vi "Create Channels from Parameter List (RT).vi"(7 "Message Param map in":T1, 8 "error in (no error)":errorcluster, 10 "Param ID map in":map{i32, string}(c390), 11 "channel ref in":T2=18446744073709551615 format="%.0x") -> (0 "error out":errorcluster, 2 "Param ID map out":map{i32, string}(c390), 3 "channel ref out":T2=18446744073709551615 format="%.0x", 5 "Message Param map out":T1)   [LabVIEW 2020, in "Ballard 1553 System Explorer.lvlib"]
uses:
  Ballard 1553 System Explorer.lvlib
  <vilib>/NI VeriStand/Custom Device API/Custom Device Item Ref.ctl
  Parse XML Ballard/Ballard_RT direction.ctl
  <vilib>/NI VeriStand/Custom Device API/Custom Device Channel Type.ctl
  Shared/Controls and Global/Global.vi
  <vilib>/NI VeriStand/Custom Device Tools/Custom Device Utility Library/NI VeriStand - Search for All Items by GUID.vi
  <vilib>/NI VeriStand/Custom Device API/Get Item Property (I32).vi
  <vilib>/NI VeriStand/Custom Device API/Get Item Property (U16).vi
  <vilib>/NI VeriStand/Custom Device Tools/Custom Device Utility Library/NI VeriStand - Search for Item by GUID.vi
  <vilib>/NI VeriStand/Custom Device Tools/Custom Device Utility Library/Custom Device Utility Library.lvlib
  Shared/Ballard 1553 Shared.lvlib
  <vilib>/NI VeriStand/Custom Device API/Custom Device API.lvlib
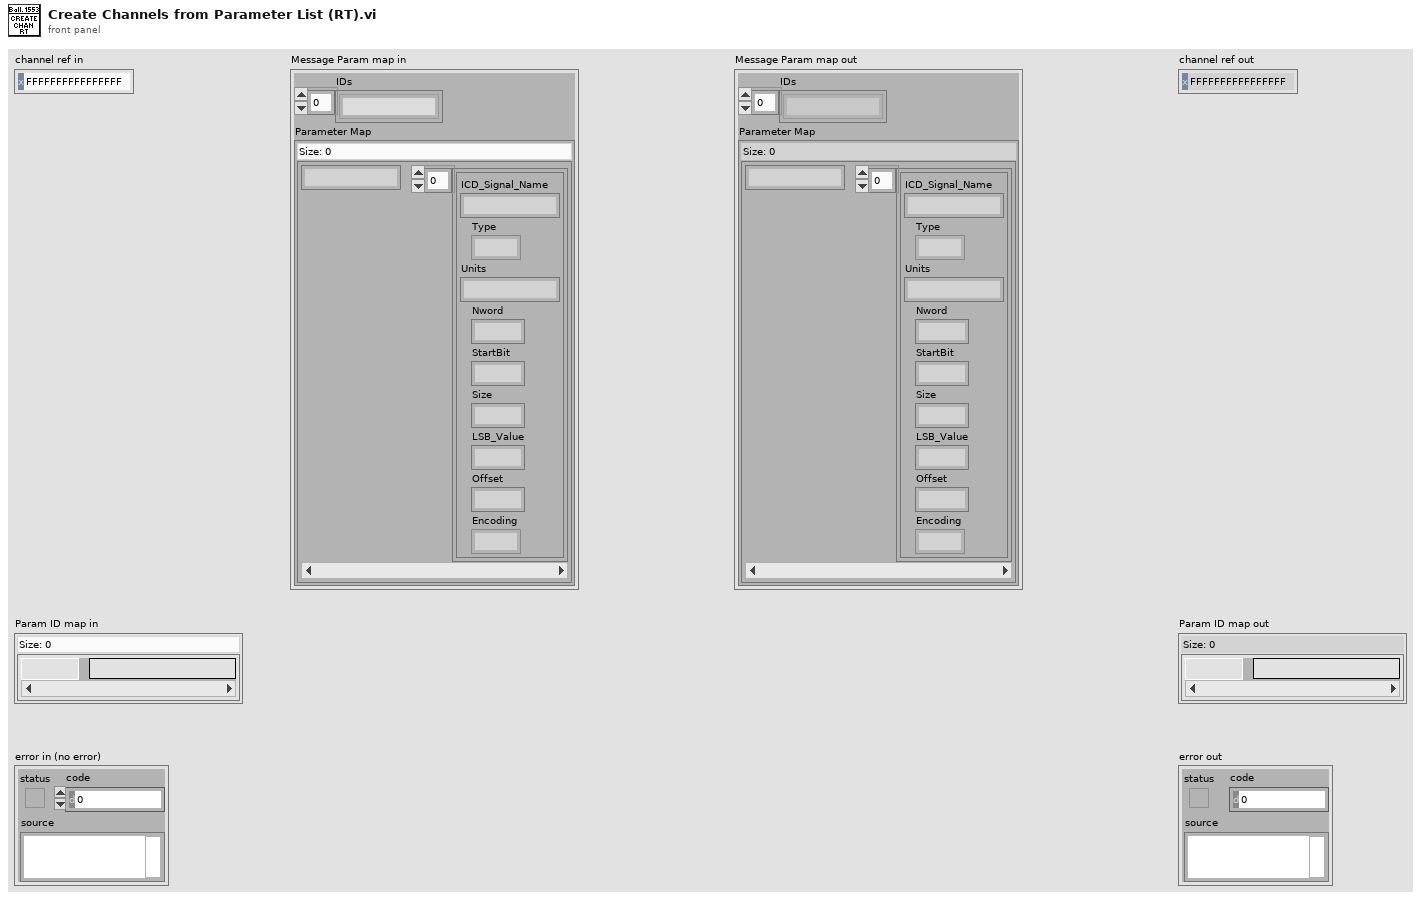
[diagram p1: front panel]
types:
  T1 = cluster{"IDs":string[], "Parameter Map":map{string, cluster{"ICD_Signal_Name":string, "Type":enum16{"Opaque", "Enum", "Float", "Integer", "Bcd", "Bool"}, "Units":string, "Nword":i32, "StartBit":i32, "Size":i32, "LSB_Value":dbl, "Offset":i32, "Encoding":enum16{"None", "2-complement", "Unsigned"}}[]}}
  T2 = typedef "Custom Device API.lvlib/Custom Device Item Ref.ctl" = u64
  T3 = typedef "Ballard 1553 System Explorer.lvlib/Ballard_RT direction.ctl" = enum16{"Tx", "Rx"}
  T4 = typedef "Custom Device API.lvlib/Custom Device Channel Type.ctl" = enum16{"Input", "Output"}
  T5 = map{string, cluster{"ICD_Signal_Name":string, "Type":enum16{"Opaque", "Enum", "Float", "Integer", "Bcd", "Bool"}, "Units":string, "Nword":i32, "StartBit":i32, "Size":i32, "LSB_Value":dbl, "Offset":i32, "Encoding":enum16{"None", "2-complement", "Unsigned"}}[]}
  T6 = cluster{"ICD_Signal_Name":string, "Type":enum16{"Opaque", "Enum", "Float", "Integer", "Bcd", "Bool"}, "Units":string, "Nword":i32, "StartBit":i32, "Size":i32, "LSB_Value":dbl, "Offset":i32, "Encoding":enum16{"None", "2-complement", "Unsigned"}}[]
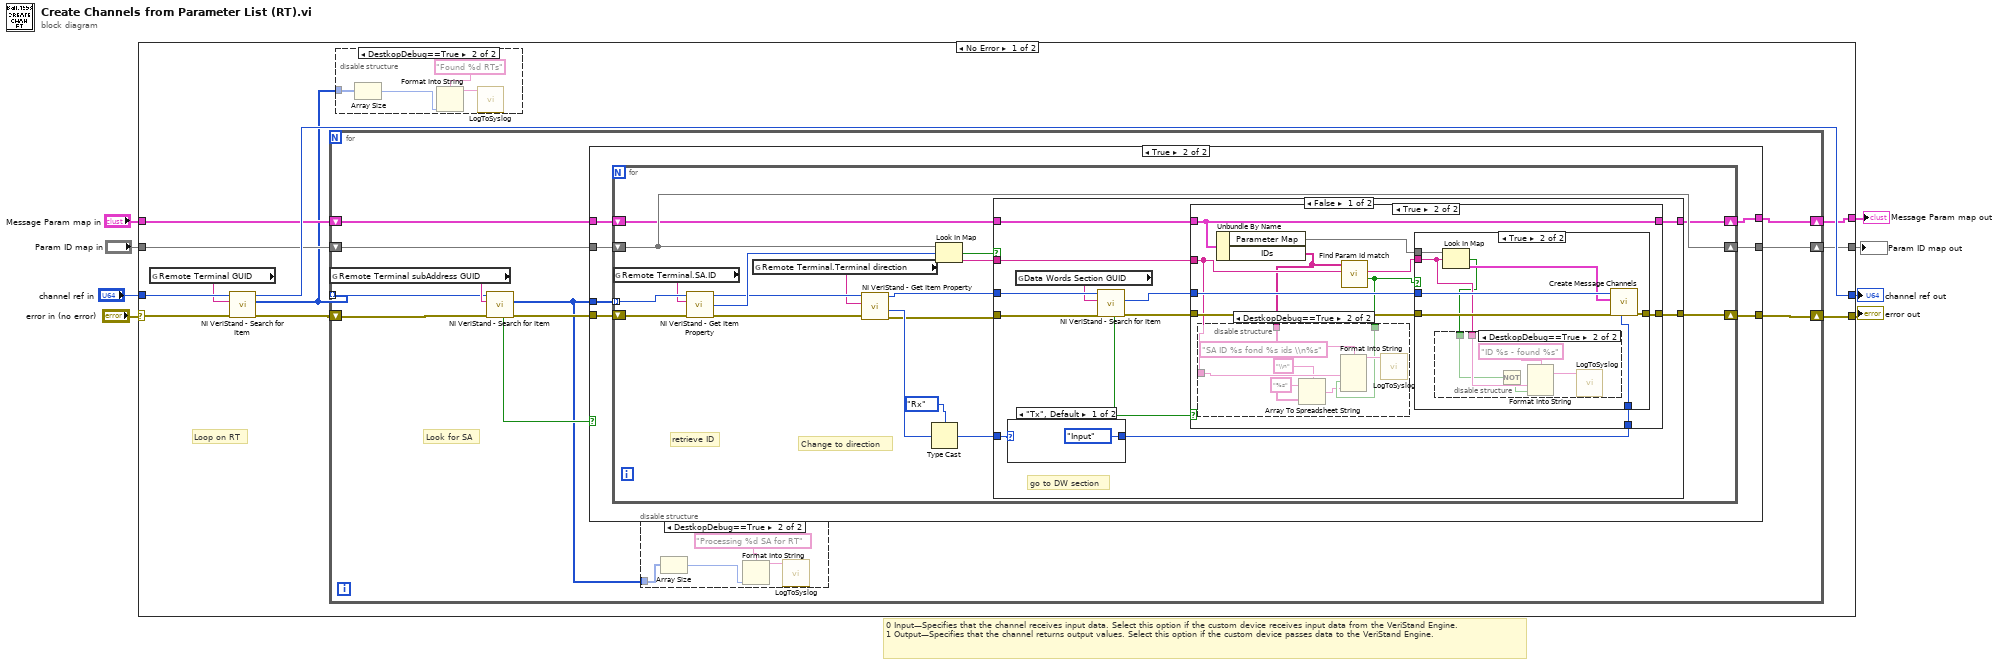
[diagram p0: block diagram]
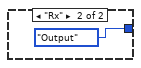
[diagram p4: hidden frame]
diagram:
  # "0 Input—Specifies that the channel receives input data. Select this option if the custom device receives input data from the VeriStand Engine. \n1 Output—Specifies that the channel returns output values. Select this option if the custom device passes data to the VeriStand Engine."
  n1 = case shown="No Error" "error in (no error)" {
    selector: "error in (no error)" -> [w18 w118]
    tunnel: "channel ref in" -> [w19 w120]
    tunnel: "Param ID map in" -> [w14 w119]
    tunnel: [w17 w120] -> w5
    tunnel: [w13 w119] -> w4
    tunnel: [w15 w118] -> w3
    tunnel: "Message Param map in" -> [w12 w117]
    tunnel: [w11 w117] -> w1
    frame No Error {
      # "Loop on RT"
      n2 = global read "Global.vi" "Remote Terminal GUID"() -> (w10:string)
      n3 = call-poly <vilib>:"NI VeriStand - Search for Item.vi"("error in"=w18, "Item GUID"=w10, "Section Ref in"=w19) -> ("error out"=w16:errorcluster, "Item Refs"=w9:T2[], "Section Ref out"=w17:T2)  [unwired: 5 in, 1 out]
      n4 = for {
        tunnel: w9 -> [w25] mode=indexing
        shift-right: [w27] -> w15
        shift-left: w16 -> [w30]
        shift-right: [w21] -> w11
        shift-left: w12 -> [w22]
        shift-right: [w23] -> w13
        shift-left: w14 -> [w24]
        # "Look for SA"
        n5 = global read "Global.vi" "Remote Terminal subAddress GUID"() -> (w29:string)
        n6 = call-poly <vilib>:"NI VeriStand - Search for Item.vi"("error in"=w30, "Item GUID"=w29, "Section Ref in"=w25) -> ("error out"=w26:errorcluster, "Item Refs"=w20:T2[], "Found"=w28:bool)  [unwired: 5 in, 1 out]
        n7 = case shown="True" w28 {
          tunnel: w20 -> [_ w44]
          tunnel: [w37 w42] -> w27
          tunnel: w26 -> [w37 w43]
          tunnel: w24 -> [w36 w41]
          tunnel: [w36 w40] -> w23
          tunnel: w22 -> [w35 w39]
          tunnel: [w35 w38] -> w21
          frame False {
          }
          frame True {
            n8 = for {
              tunnel: w44 -> [w60] mode=indexing
              shift-right: [w62] -> w42
              shift-left: w43 -> [w61]
              shift-right: [w58] -> w40
              shift-left: w41 -> [w58]
              shift-right: [w53] -> w38
              shift-left: w39 -> [w54]
              # "Change to direction"
              # "retrieve ID"
              n9 = global read "Global.vi" "Remote Terminal.SA.ID"() -> (w59:string)
              n10 = call-poly <vilib>:"NI VeriStand - Get Item Property.vi"("error in (no error)"=w61, "Property Name"=w59, "Item Ref in"=w60) -> ("error out"=w51:errorcluster, "Value"=w57:i32, "Item Ref out"=w52:T2)  [unwired: 5 in, 1 out]
              n11 = global read "Global.vi" "Remote Terminal.Terminal direction"() -> (w46:string)
              n12 = call-poly <vilib>:"NI VeriStand - Get Item Property.vi"("error in (no error)"=w51, "Property Name"=w46, "Item Ref in"=w52) -> ("error out"=w49:errorcluster, "Value"=w50:u16, "Item Ref out"=w48:T2)  [unwired: 5 in, 1 out]
              n13 = Type Cast(type=Ballard_RT_direction."Rx" ("y"), x=w50) -> (*(type *) &x=w47:T3)
              n14 = Look In Map(map=w58, key=w57) -> (key not found?=w56:bool, value=w55:string)  [unwired: 1 in]
              n15 = case shown="False" w56 {
                tunnel: [w69 w112] -> w62
                tunnel: w48 -> [w74 _]
                tunnel: w49 -> [w73 w112]
                tunnel: w55 -> [w63 _]
                tunnel: w54 -> [w68 w111]
                tunnel: [w67 w111] -> w53
                tunnel: w47 -> [w65 _]
                frame False {
                  # "go to DW section"
                  n16 = case shown="\"Tx\", Default" w65 {
                    tunnel: [Custom_Device_Channel_Type."Input" ("VS channel direction") Custom_Device_Channel_Type."Output" ("VS channel direction")] -> w64
                    frame "Tx", Default {
                    }
                    frame "Rx" {
                    }
                  }
                  n17 = global read "Global.vi" "Data Words Section GUID"() -> (w66:string)
                  n18 = call-poly <vilib>:"NI VeriStand - Search for Item.vi"("error in"=w73, "Item GUID"=w66, "Section Ref in"=w74) -> ("error out"=w72:errorcluster, "Item Ref"=w71:T2, "Found"=w70:bool)  [unwired: 5 in, 1 out]
                  n19 = case shown="True" w70 {
                    tunnel: w72 -> [w77 w88]
                    tunnel: w71 -> [_ w87]
                    tunnel: [w77 w86] -> w69
                    tunnel: w68 -> [w78 w84]
                    tunnel: [w78 w84] -> w67
                    tunnel: w64 -> [_ w85]
                    tunnel: w63 -> [_ w81]
                    frame False {
                    }
                    frame True {
                      n20 = Unbundle By Name(w84) -> ("Parameter Map"=w83:T5, "IDs"=w80:string[])
                      n21 = call "Find Param Id match.vi"("RT partial Id in"=w81, "Id List in"=w80) -> ("found"=w79:bool, "Matched id out"=w82:string)  [unwired: 7 in, 1 out]
                      n22 = disable-structure shown="DestkopDebug==True" {
                        disable-tunnel: w81 -> [_ w94]
                        disable-tunnel: w80 -> [_ w93]
                        disable-tunnel: w79 -> [_ w91]
                        frame condition #0 (active) {
                        }
                        frame condition #1 {
                          n23 = Array To Spreadsheet String(delimiter (Tab)="\\n", array=w93, 3:"%s" ("format string")) -> (spreadsheet string=w90:string)
                          n24 = Format Into String(format string="SA ID %s fond %s ids \\n%s", w94, w91, w90) -> (resulting string=w95:string)  [unwired: 2 in, 1 out]
                          n25 = call "LogToSyslog.vi"("message"=w95) -> ()  [unwired: 9 in, 2 out]
                        }
                      }
                      n26 = case shown="True" w79 {
                        tunnel: w88 -> [w97 w105]
                        tunnel: w87 -> [_ w104]
                        tunnel: [w97 w103] -> w86
                        tunnel: w85 -> [_ w102]
                        tunnel: w83 -> [_ w101]
                        tunnel: w82 -> [_ w99]
                        frame False {
                        }
                        frame True {
                          n27 = Look In Map(map=w101, key=w99) -> (key not found?=w98:bool, value=w100:T6)  [unwired: 1 in]
                          n28 = disable-structure shown="DestkopDebug==True" {
                            disable-tunnel: w99 -> [_ w108]
                            disable-tunnel: w98 -> [_ w107]
                            frame condition #0 (active) {
                            }
                            frame condition #1 {
                              n29 = Not(x=w107) -> (.not. x?=w106:bool)
                              n30 = Format Into String(format string="ID %s - found %s", w108, w106) -> (resulting string=w109:string)  [unwired: 2 in, 1 out]
                              n31 = call "LogToSyslog.vi"("message"=w109) -> ()  [unwired: 9 in, 2 out]
                            }
                          }
                          n32 = call "Create Message Channels.vi"("VS channel direction"=w102, "error in (no error)"=w105, "Parameters"=w100, "Data Words section in"=w104) -> ("error out"=w103:errorcluster)  [unwired: 6 in, 1 out]
                        }
                      }
                    }
                  }
                }
                frame True {
                }
              }
            }
          }
        }
        n33 = disable-structure shown="DestkopDebug==True" {
          disable-tunnel: w20 -> [_ w33]
          frame condition #0 (active) {
          }
          frame condition #1 {
            n34 = Array Size(array=w33) -> (size(s)=w32:i32)
            n35 = Format Into String(format string="Processing %d SA for RT", w32) -> (resulting string=w31:string)  [unwired: 2 in, 1 out]
            n36 = call "LogToSyslog.vi"("message"=w31) -> ()  [unwired: 9 in, 2 out]
          }
        }
      }
      n37 = disable-structure shown="DestkopDebug==True" {
        disable-tunnel: w9 -> [_ w113]
        frame condition #0 (active) {
        }
        frame condition #1 {
          n38 = Array Size(array=w113) -> (size(s)=w115:i32)
          n39 = Format Into String(format string="Found %d RTs", w115) -> (resulting string=w114:string)  [unwired: 2 in, 1 out]
          n40 = call "LogToSyslog.vi"("message"=w114) -> ()  [unwired: 9 in, 2 out]
        }
      }
    }
    frame Error {
    }
  }
  "error out" <- w3
  "channel ref out" <- w5
  "Param ID map out" <- w4
  "Message Param map out" <- w1
